vi "AbortSingle.vi"(8 "error in (no error)":errorcluster, 10 "axis name? (all)":string, 11 "controller in":refnum<k24>) -> (0 "error out":errorcluster, 3 "controller out":refnum<k24>)   [LabVIEW 2016]
uses:
  C:/user/patrick/git/Aerotech-Delay-Line/lvsrc/Aerotech-Ensemble-LabVIEW/8.2/Bin/Aerotech.Ensemble.dll
  Bin/Aerotech.Ensemble.dll
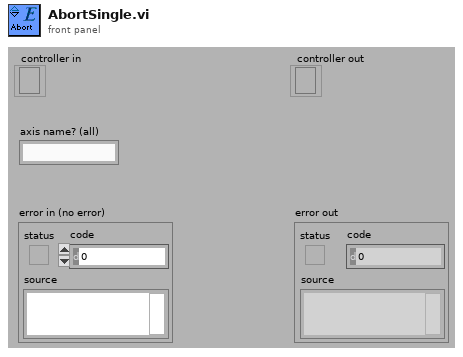
[diagram p1: front panel]
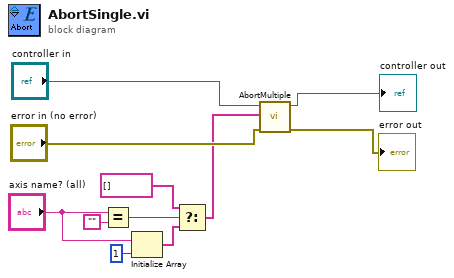
[diagram p0: block diagram]
diagram:
  n1 = Equal?(x="axis name? (all)", y="") -> (x = y?=w6:bool)
  n2 = Initialize Array("axis name? (all)", 1 ("dimension size")) -> (w3:string[])
  n3 = Select(t=string[] [] ("initialized array"), s=w6, f=w3) -> (s? t:f=w4:string[])
  n4 = call "AbortMultiple.vi"("error in (no error)"="error in (no error)", "axis names"=w4, "controller in"="controller in") -> ("error out"=→"error out":errorcluster, "controller out"=→"controller out":refnum<k24>)  [unwired: 7 in]
